vi "Terminal-DriverSystem-ParametersSetter.vi"(8 "error in (no error)":errorcluster caption="错误输入（无错误）", 10 "转速":u16, 11 "write operation timeout (ms)":i32=5000 caption="写操作超时（5000毫秒）") -> (0 "error out":errorcluster caption="错误输出")   [LabVIEW 2014]
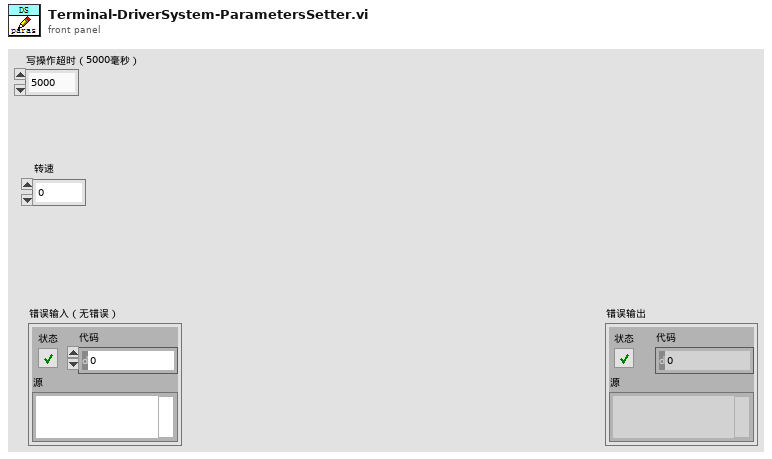
[diagram p1: front panel]
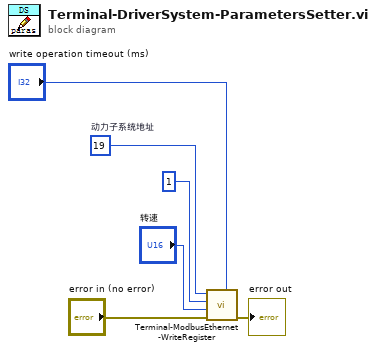
[diagram p0: block diagram]
diagram:
  w3 = u8 19  # 动力子系统地址
  n1 = call "Terminal-ModbusEthernet-WriteRegister.vi"("write operation timeout (ms)"="write operation timeout (ms)", "error in"="error in (no error)", "holding register value"="转速", "address"=u16 1, "unit ID"=w3) -> ("error out"=→"error out":errorcluster)  [unwired: 6 in]
